vi "ModeFromDevices.vi"(8 "error in (no error)":errorcluster, 10 "Devices queue":refnum<queue>) -> (0 "error out":errorcluster, 2 "Mode Col":i32)   [LabVIEW 2013]
uses:
  Device/Device.lvclass
  Master Device/Master Device.lvclass
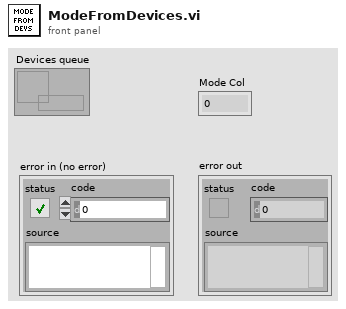
[diagram p1: front panel]
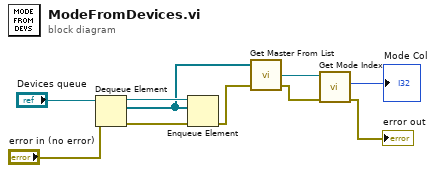
[diagram p0: block diagram]
diagram:
  n1 = Dequeue Element(queue="Devices queue", error in (no error)="error in (no error)") -> (queue out=w8:refnum<queue>, element=w6:refnum<class "Device.lvclass">[], error out=w7:errorcluster)  [unwired: 1 in, 1 out]
  n2 = Enqueue Element(queue=w8, element=w6, error in (no error)=w7) -> (error out=w5:errorcluster)  [unwired: 1 in, 2 out]
  n3 = call "Get Master From List.vi"("error in"=w5, "Device List in"=w6) -> ("error out"=w9:errorcluster, "Master Device"=w10:refnum<class "Master Device.lvclass">)  [unwired: 1 in, 1 out]
  n4 = call-dynamic "Get Mode Index.vi"("error in (no error)"=w9, "Master Device in"=w10) -> ("error out"=→"error out":errorcluster, "Mode Col"=→"Mode Col":i32)  [unwired: 7 in, 1 out]
